vi "Receiver_Example_Image.vi"() -> ()   [LabVIEW 2018]
panel:
  out "error out 2":errorcluster
  out "data":cluster{"t0":dbl, "dt":dbl, "Y":cdb[]}
  out "size(s) 3":i32
  out "output array":i8[](array[numeric])
  in  "array":i8[](array[numeric])
  out "sisa bagi":i32
  out "hasil bagi":i32
  out "iterasi":i32
  out "size(s) 2":i32
  out "output bit stream 2":i8[](array[numeric]) caption="output bit stream"
  in  "path to BMP file 2":path
  in  "Numeric":i32
  out "BER":dbl
  out "SNR":dbl
  in  "Modulation parameter":T1
  out "created new?":bool
  out "SIG valid?":bool
  in  "stop":bool
  out "USRP CoercedParamters":T2={"coerced IQ rate"=100000.0, "coerced carrier frequency"=100000.0, "coerced gain"=0.0} {"coerced gain" format="%#_6f"; "coerced carrier frequency" format="%#_6p"; "coerced IQ rate" format="%#_6p"}
  out "error out":errorcluster
  in  "Trigger level":dbl=0.005 format="%f"
  in  "error in (no error)":errorcluster
  in  "USRP ControledParameters":T3={"active antenna"="RX1", "gain"=0.0, "carrier frequency"=915000000.0, "IQ rate"=1000000.0} {"IQ rate" format="%#_6p"; "carrier frequency" format="%#_6p"; "gain" format="%#_6f"}
  in  "device names":refnum<k15>="192.168.10.4"
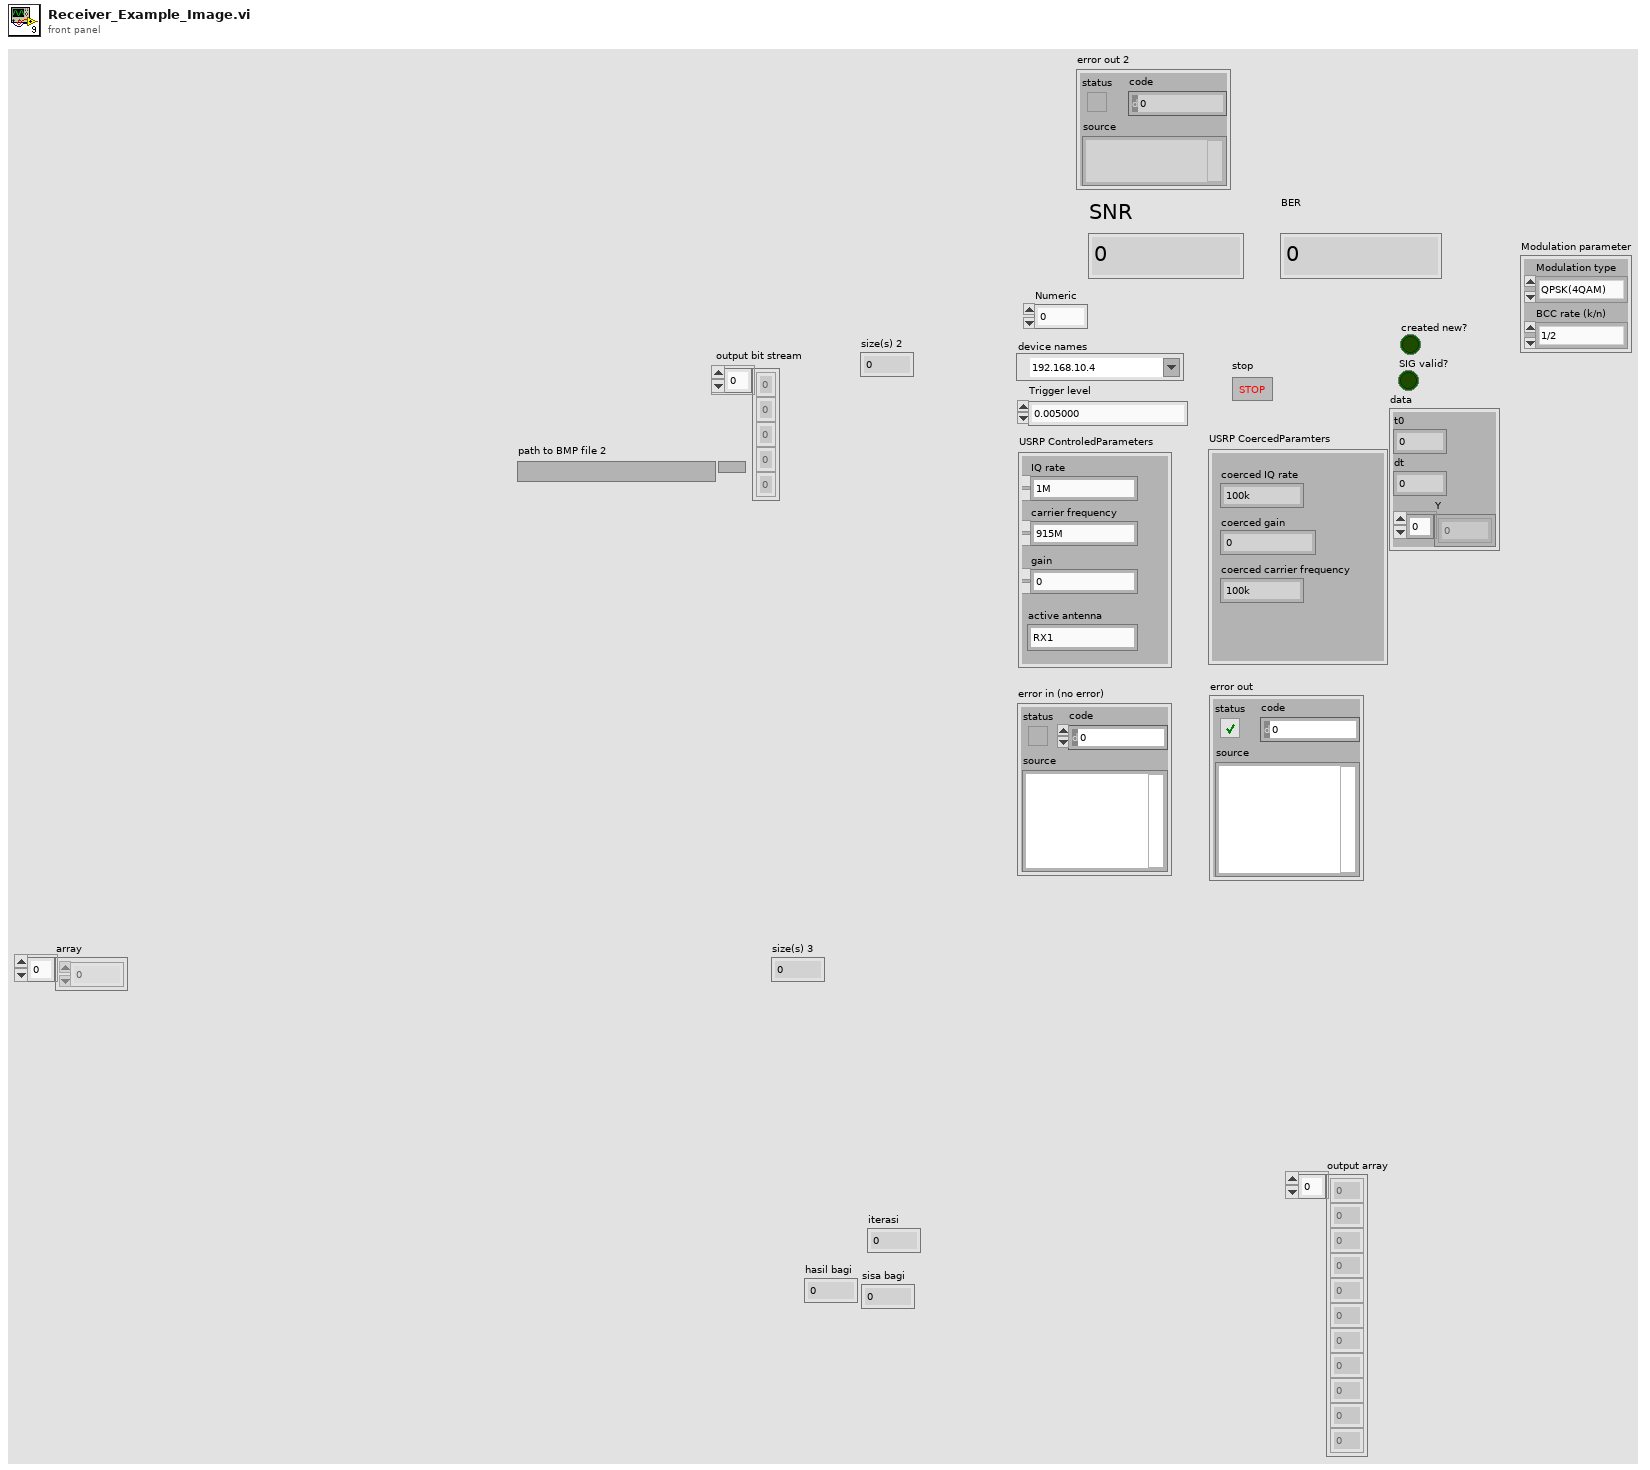
[diagram p1: front panel]
types:
  T1 = cluster{"Modulation type":enum16{"QPSK(4QAM)", "64QAM", "16QAM", "BPSK"}, "BCC rate (k/n)":enum16{"1/2", "2/3", "3/4"}}
  T2 = cluster{"coerced IQ rate":dbl, "coerced carrier frequency":dbl, "coerced gain":dbl}
  T3 = cluster{"active antenna":string, "gain":dbl, "carrier frequency":dbl, "IQ rate":dbl}
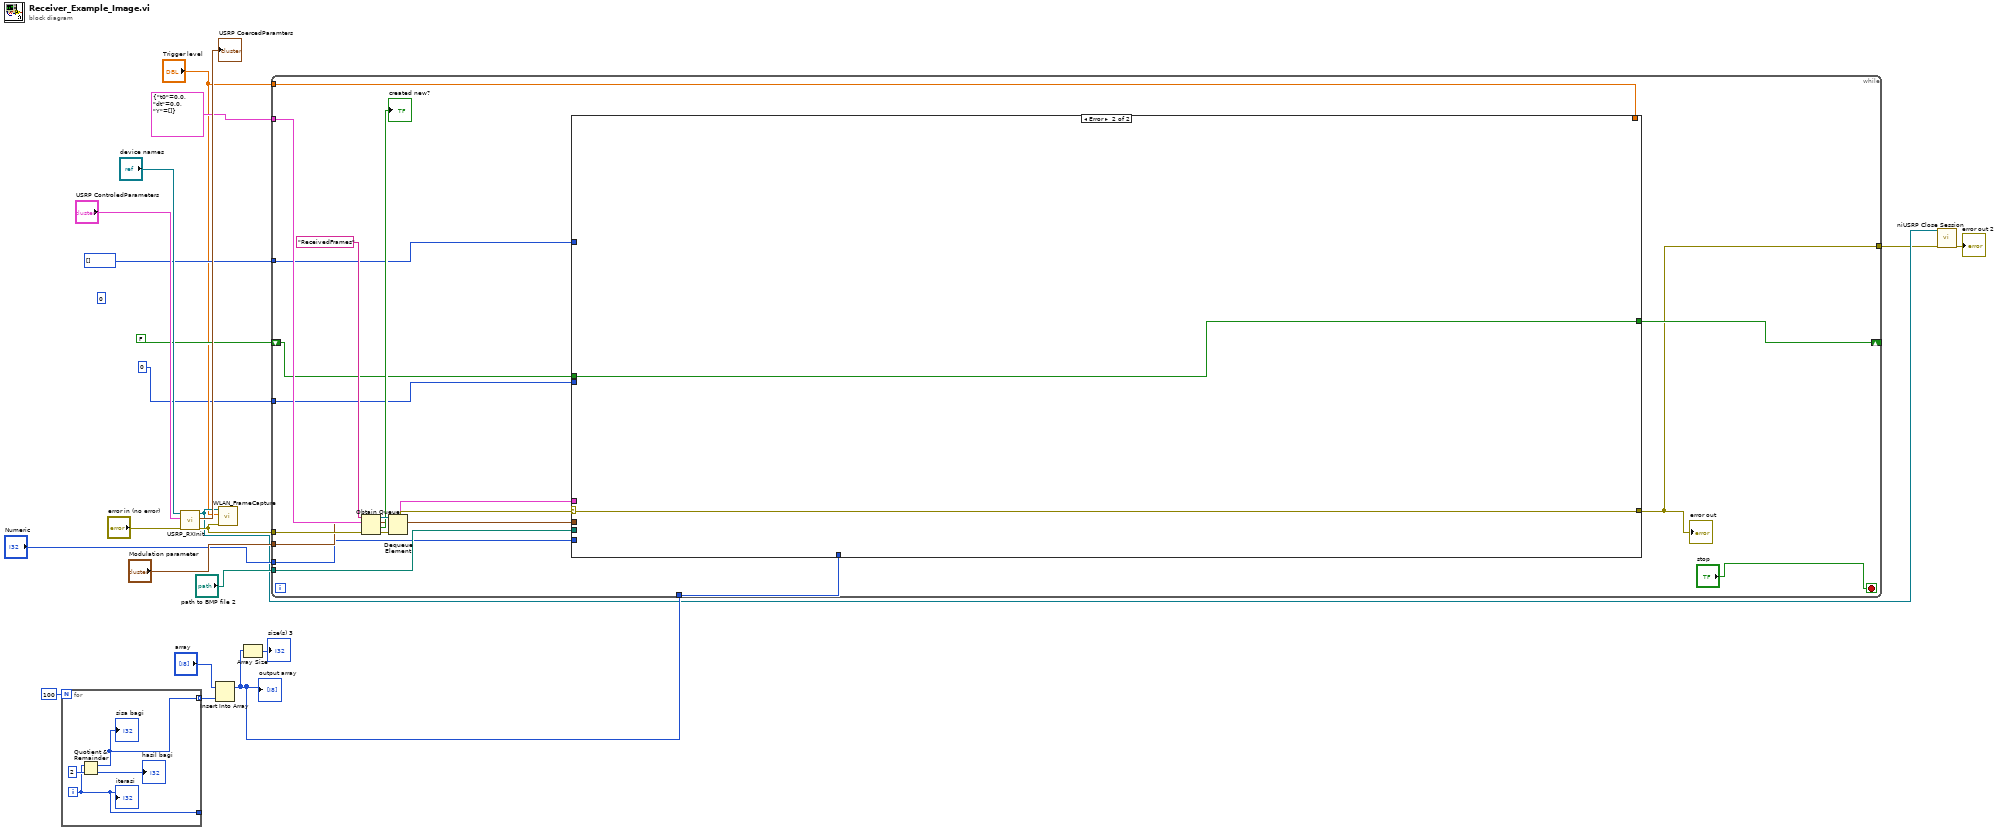
[diagram p0: block diagram]
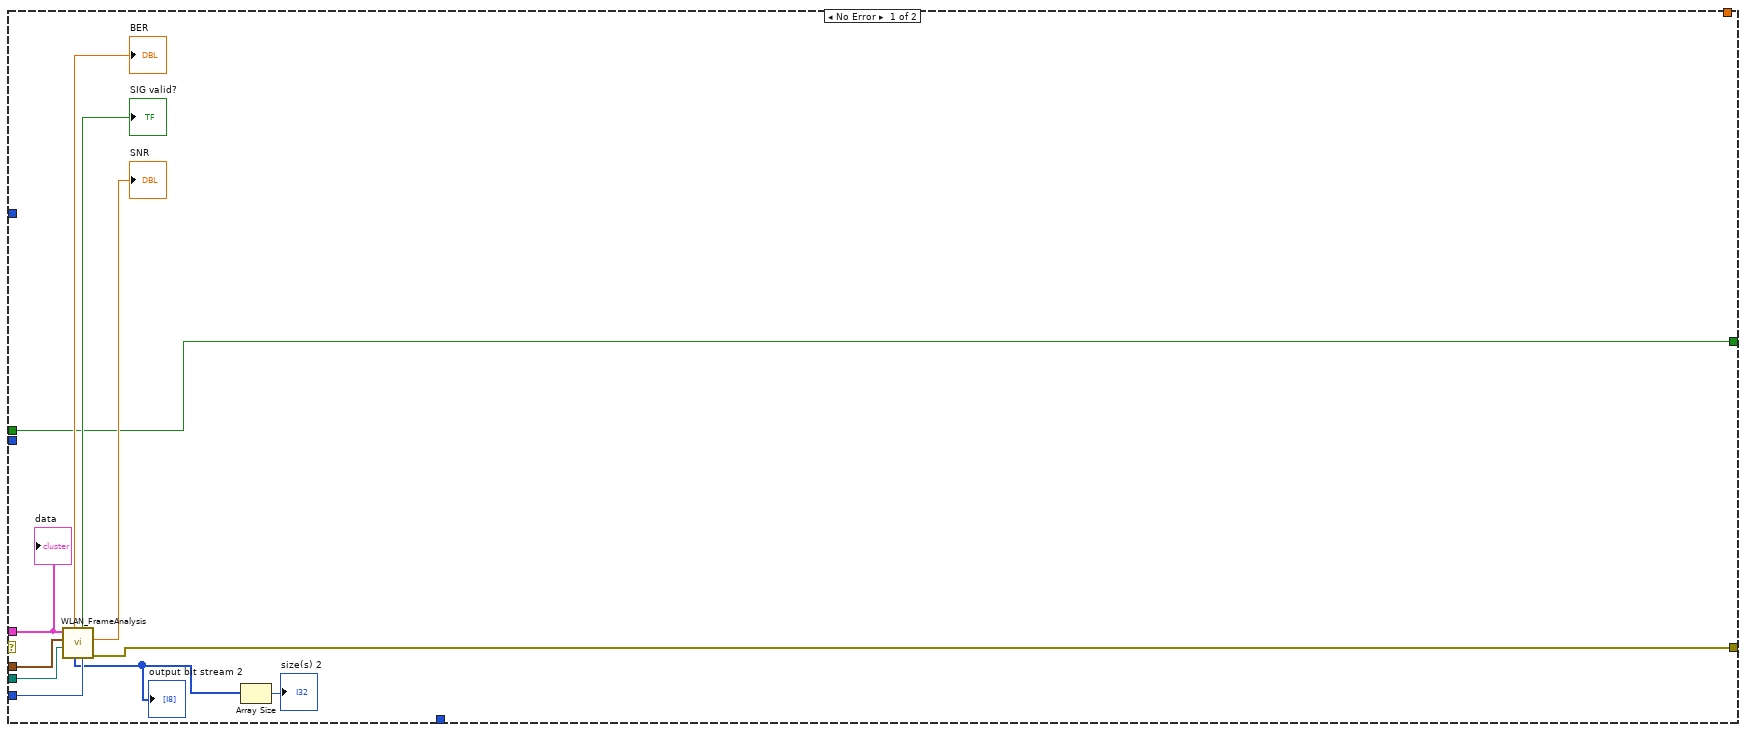
[diagram p2: hidden frame]
diagram:
  (unwired) 0
  n1 = for {
    N: 100 -> [_]
    tunnel: [w23] -> _
    tunnel: [w22] -> w11 mode=indexing
    i -> [w23]
    n2 = Quotient & Remainder(x=w23, y=2) -> (x-y*floor(x/y)=w22:i32, floor(x/y)=→"hasil bagi":i32)
    "sisa bagi" <- w22
    "iterasi" <- w23
  }
  n3 = call "USRP_RXInit.vi"("device names"="device names", "USRP ControledParameters"="USRP ControledParameters", "error in (no error)"="error in (no error)") -> ("session handle out"=w6:refnum<k15>, "USRP CoercedParamters"=→"USRP CoercedParamters":T2, "error out"=w17:errorcluster)  [unwired: 5 in]
  n4 = Insert Into Array(array="array", new element=w11) -> (w8:i8[])  [unwired: 1 in]
  "output array" <- w8
  n5 = call "WLAN_FrameCapture.vi"("error in (no error)"=w17, "Trigger level"="Trigger level", "session handle"=w6) -> ()  [unwired: 8 in]
  n6 = Array Size(array=w8) -> (size(s)=→"size(s) 3":i32)
  n7 = while {
    tunnel: w17 -> [w43]
    tunnel: cluster{"t0":dbl, "dt":dbl, "Y":cdb[]} {"t0"=0.0, "dt"=0.0, "Y"=[]} ("data") -> [w44]
    tunnel: "Modulation parameter" -> [w36]
    tunnel: "path to BMP file 2" -> [w35]
    tunnel: "Numeric" -> [w34]
    tunnel: w8 -> [w33]
    shift-right: [w31] -> _
    shift-left: FALSE ("x = y?") -> [w32]
    tunnel: i32[] [] -> [w29]
    tunnel: "Trigger level" -> [w28]
    tunnel: 0 -> [w27]
    tunnel: [w26] -> w2
    stop <- "stop" stop-if-true
    n8 = Obtain Queue(name (unnamed)="ReceivedFrames", element data type=w44, error in (no error)=w43) -> (queue out=w42:refnum<queue>, created new?=→"created new?":bool, error out=w39:errorcluster)  [unwired: 2 in]
    n9 = Dequeue Element(queue=w42, error in (no error)=w39) -> (element=w40:cluster{"t0":dbl, "dt":dbl, "Y":cdb[]}, error out=w41:errorcluster)  [unwired: 1 in, 2 out]
    n10 = case shown="Error" w41 {
      selector: w41 -> [_ w57]
      tunnel: w40 -> [w53 _]
      tunnel: [w54 w57] -> w26
      tunnel: w36 -> [w52 _]
      tunnel: w35 -> [w48 _]
      tunnel: w34 -> [w49 _]
      tunnel: w33 -> [_ _]
      tunnel: w32 -> [w45 w56]
      tunnel: [w45 w56] -> w31
      tunnel: w29 -> [_ _]
      tunnel: w28 -> [_ _]
      tunnel: w27 -> [_ _]
      frame No Error {
        n11 = call "WLAN_FrameAnalysis.vi"("Numeric"=w49, "path to BMP file"=w48, "Modulation parameter"=w52, "input cluster"=w53) -> ("error out"=w54:errorcluster, "SNR"=→"SNR":dbl, "SIG valid?"=→"SIG valid?":bool, "output bit stream 2"=w46:i8[], "BER"=→"BER":dbl)  [unwired: 1 in, 2 out]
        "output bit stream 2" <- w46
        n12 = Array Size(array=w46) -> (size(s)=→"size(s) 2":i32)
        "data" <- w53
      }
      frame Error {
      }
    }
    "error out" <- w26
  }
  n13 = call <instrlib>:"niUSRP Close Session.vi"("session handle"=w6, "error in (no error)"=w2) -> ("error out"=→"error out 2":errorcluster)  [unwired: 13 in]
